vi "Is VI Server Required.vi"(8 "error in (no error)":errorcluster, 11 "Mouse Action in":refnum<class "Mouse Action.lvclass">) -> (0 "error out":errorcluster, 2 "VI Server Required?":bool, 3 "Mouse Action out":refnum<class "Mouse Action.lvclass">)   [LabVIEW 2020, in "MacroAssert.lvlib" / "Mouse Action.lvclass"]
doc: "Outputs whether VI Server is required to perform the given step."
uses:
  Mouse Action.lvclass
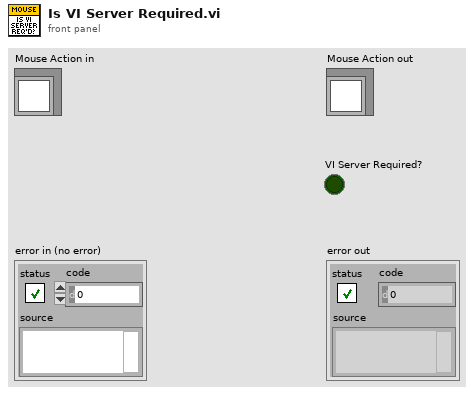
[diagram p1: front panel]
types:
  T1 = typedef "MacroAssert.lvlib/Mouse Action.lvclass/Mouse Action Type.ctl" = enum16{"Click", "Absolute Move", "Absolute Move and Click", "Relative Move", "Relative Move and Click", "Wheel Up", "Wheel Down"}
  T2 = typedef "MacroAssert.lvlib/Mouse Action.lvclass/Relative Movement Type.ctl" = enum16{"Pixels from Current Position", "Pixels from Top-Left of Control", "Pixels from Top-Left of Window", "Percentage from Top-Left of Control", "Percentage from Top-Left of Window", "Percentage from Top-Left of Screen"}
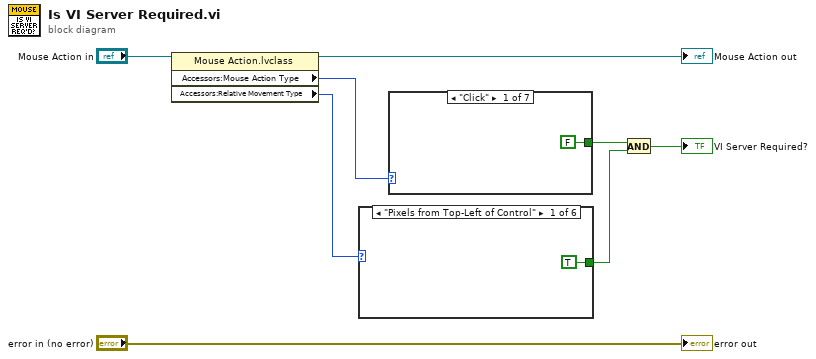
[diagram p0: block diagram]
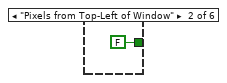
[diagram p2: hidden frame]
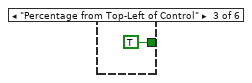
[diagram p3: hidden frame]
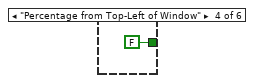
[diagram p4: hidden frame]
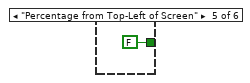
[diagram p5: hidden frame]
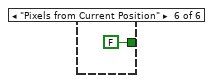
[diagram p6: hidden frame]
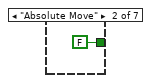
[diagram p7: hidden frame]
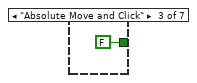
[diagram p8: hidden frame]
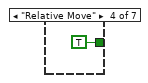
[diagram p9: hidden frame]
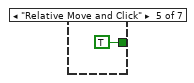
[diagram p10: hidden frame]
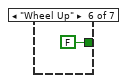
[diagram p11: hidden frame]
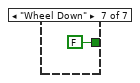
[diagram p12: hidden frame]
diagram:
  n1 = property class="Mouse Action.lvclass"(reference="Mouse Action in") -> (reference out=→"Mouse Action out":refnum<class "Mouse Action.lvclass">, "Accessors:Mouse Action Type"=w7:T1, "Accessors:Relative Movement Type"=w4:T2)  [unwired: 1 in, 1 out]
  n2 = case shown="\"Pixels from Top-Left of Control\"" w4 {
    tunnel: [TRUE FALSE TRUE FALSE FALSE FALSE] -> w2
    frame "Pixels from Top-Left of Control" {
    }
    frame "Pixels from Top-Left of Window" {
    }
    frame "Percentage from Top-Left of Control" {
    }
    frame "Percentage from Top-Left of Window" {
    }
    frame "Percentage from Top-Left of Screen" {
    }
    frame "Pixels from Current Position" {
    }
  }
  n3 = case shown="\"Click\"" w7 {
    tunnel: [FALSE FALSE FALSE TRUE TRUE FALSE FALSE] -> w1
    frame "Click" {
    }
    frame "Absolute Move" {
    }
    frame "Absolute Move and Click" {
    }
    frame "Relative Move" {
    }
    frame "Relative Move and Click" {
    }
    frame "Wheel Up" {
    }
    frame "Wheel Down" {
    }
  }
  n4 = And(x=w1, y=w2) -> (x .and. y?=→"VI Server Required?":bool)
  "error out" <- "error in (no error)"
